vi "Write Waveform as 2D Numpy Array.vi"(3 "error in":errorcluster, 4 "Waveform":waveform(dbl), 5 "Path":path) -> (0 "error out":errorcluster)   [LabVIEW 2013, in "PyLab.lvlib"]
uses:
  PyLab.lvlib
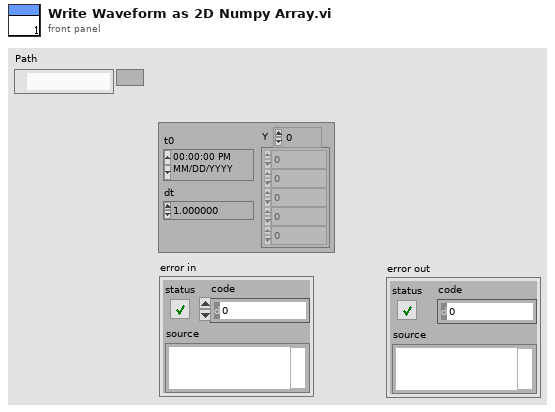
[diagram p1: front panel]
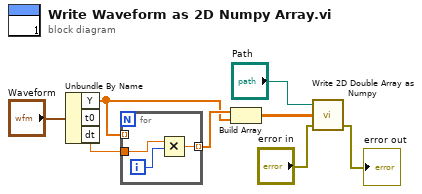
[diagram p0: block diagram]
diagram:
  n1 = Unbundle By Name("Waveform") -> ("Y"=w5:dbl[], "dt"=w7:dbl)  [unwired: 1 out]
  n2 = for {
    tunnel: w5 -> [_] mode=indexing
    tunnel: w7 -> [w10]
    tunnel: [w9] -> w6 mode=indexing
    i -> [w11]
    n3 = Multiply(x=w10, y=w11) -> (x*y=w9:dbl)
  }
  n4 = Build Array(w6, w5) -> (w4:dbl[][])
  n5 = call "Write 2D Double Array as Numpy.vi"("error in"="error in", "Array"=w4, "Path"="Path") -> ("error out"=→"error out":errorcluster)  [unwired: 2 in]
